vi "Gif.LocalColorTable.vi"(0 "data":string, 9 "offset":i32, 11 "error in (no error)":errorcluster, 12 "ImageDescriptor":T1) -> (4 "data out":string, 6 "local color table":u32[](array[numeric]), 10 "offset out":i32, 15 "error out":errorcluster)   [LabVIEW 2011]
uses:
  Gif.ImageDescriptor.ctl
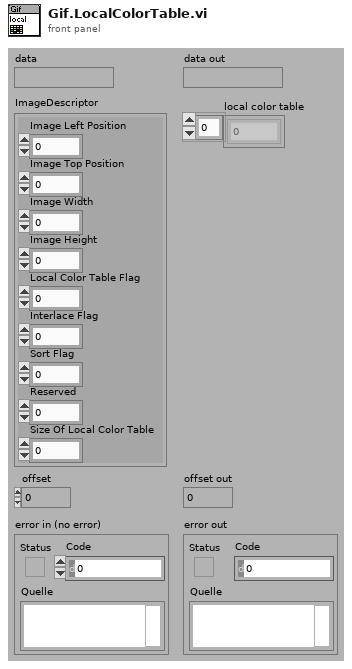
[diagram p1: front panel]
types:
  T1 = typedef "Gif.ImageDescriptor.ctl" = cluster{"Image Left Position":u16, "Image Top Position":u16, "Image Width":u16, "Image Height":u16, "Local Color Table Flag":u8, "Interlace Flag":u8, "Sort Flag":u8, "Reserved":u8, "Size Of Local Color Table":u8}
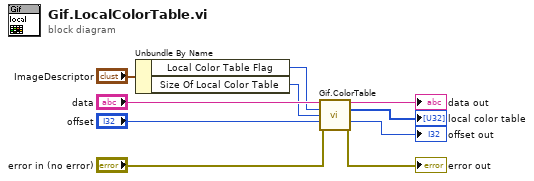
[diagram p0: block diagram]
diagram:
  n1 = Unbundle By Name("ImageDescriptor") -> ("Local Color Table Flag"=w3:u8, "Size Of Local Color Table"=w2:u8)
  n2 = call "Gif.ColorTable.vi"("data"="data", "flag"=w3, "Size of Color Table"=w2, "offset"="offset", "error in (no error)"="error in (no error)") -> ("data out"=→"data out":string, "color table"=→"local color table":u32[], "offset out"=→"offset out":i32, "error out"=→"error out":errorcluster)  [unwired: 7 out]
